vi "Kicker Pull Back.vi"(0 "Puck Energy Requirement (mJ)":dbl, 5 "Current Angle (°)":dbl, 11 "error in (no error)":errorcluster) -> (4 "Motor ON/OFF":bool, 6 "Motor FWD/RVS":bool, 8 "Puck Output Velocity":dbl, 10 "Solenoid ON/OFF":bool, 15 "error out":errorcluster)   [LabVIEW 2017]
panel:
  in  "stop":bool
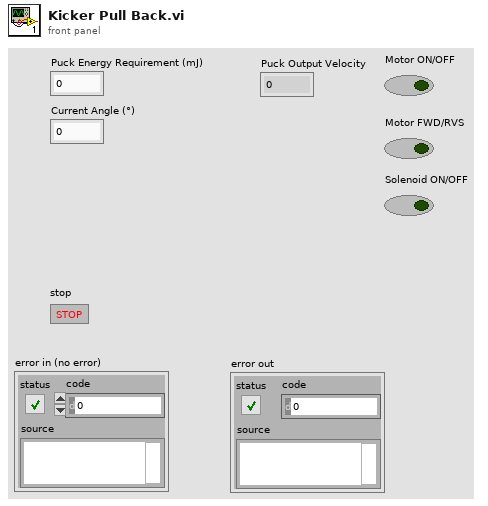
[diagram p1: front panel]
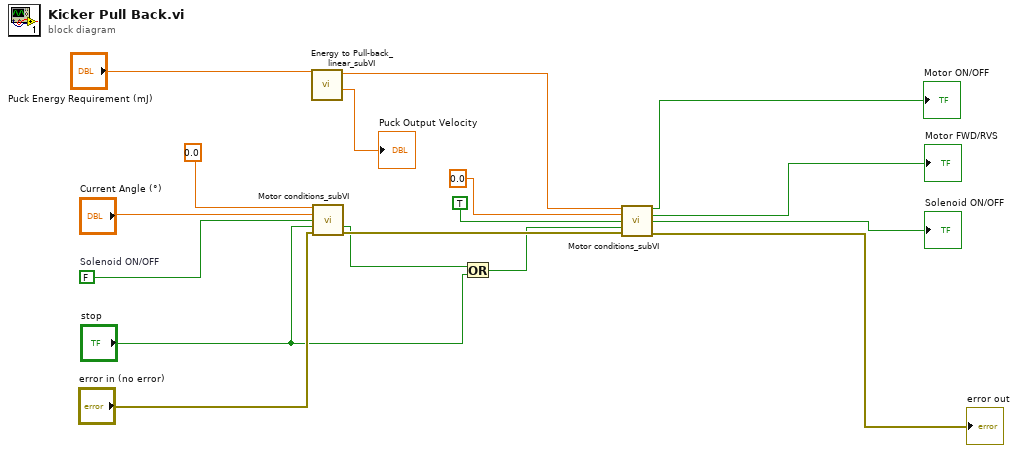
[diagram p0: block diagram]
diagram:
  w15 = FALSE  # Solenoid ON/OFF
  n1 = call "Energy to Pull-back_linear_subVI.vi"("Puck Energy Requirement (mJ)"="Puck Energy Requirement (mJ)") -> ("Output Velocity"=→"Puck Output Velocity":dbl, "Pull-back angle (°)"=w5:dbl)  [unwired: 8 in, 1 out]
  n2 = call "Motor conditions_subVI.vi"("Target Angle (°)"=0.0, "Current Angle (°)"="Current Angle (°)", "Solenoid ON/OFF"=w15, "Stop"="stop", "error in (no error)"="error in (no error)") -> ("STOP"=w3:bool, "error out"=w14:errorcluster)  [unwired: 6 in, 3 out]
  n3 = Or(x=w3, y="stop") -> (x .or. y?=w1:bool)
  n4 = call "Motor conditions_subVI.vi"("Target Angle (°)"=w5, "Current Angle (°)"=0.0, "Solenoid ON/OFF"=TRUE, "Stop"=w1, "error in (no error)"=w14) -> ("Motor On/Off"=→"Motor ON/OFF":bool, "Motor FWD/RVS"=→"Motor FWD/RVS":bool, "Solenoid ON/OFF"=→"Solenoid ON/OFF":bool, "error out"=→"error out":errorcluster)  [unwired: 6 in, 1 out]
